vi "RAMP_init_ramp_scan.vi"(0 "queue CAMERA":refnum<queue>, 1 "queue piezo":refnum<queue>, 2 "queue DAQ":refnum<queue>, 3 "queue ASI stage":refnum<queue>, 4 "Laser lines array":dbl[][](array[numeric]), 5 "error in":errorcluster, 6 "Illumination source":bool, 7 "Brightfield intensity":dbl, 8 "Autofocus":bool, 9 "Movie path":path, 10 "Total range (nm)":u32=2000, 11 "z step (nm)":u32=50, 12 "Start acquisition":bool, 13 "Exp time (s)":sgl=0.05 format="%#_3g") -> (14 "Ramp":dbl[](array[numeric]), 16 "Total # z steps":i32, 17 "Ready":bool, 19 "error out":errorcluster)   [LabVIEW 2015]
uses:
  CONTROLS/Q_MCL_piezo_element.ctl
  CONTROLS/Q_camera_element.ctl
  CONTROLS/Q_ASI_stage_element.ctl
  CONTROLS/Q_DAQ_element.ctl
  GLOBAL/Global_DAQ.vi
  GLOBAL/Global_ASI_stage.vi
  GLOBAL/Global_MCL_piezo.vi
  GLOBAL/Global_CAMERA.vi
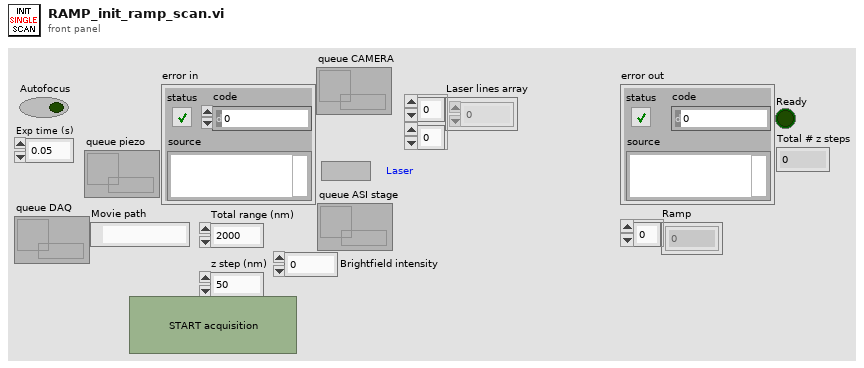
[diagram p1: front panel]
types:
  T1 = cluster{"Frames":i32, "Movie path":path, "Start acquisition":bool}
  T2 = typedef "Q_DAQ_element.ctl" = cluster{"variant":variant, "Instruction":enum16{"DAQ_idle", "DAQ_initialize", "DAQ_error", "DAQ_security_stop", "DAQ_start_QPD", "DAQ_change_QPD_display", "DAQ_read_display_QPD_signal", "DAQ_QPD_init_autofocus", "DAQ_read_display_send_QPD_signal", "DAQ_close_autofocus_calibration_ramp", "DAQ_close_autofocus", "DAQ_405", "DAQ_488", "DAQ_561", "DAQ_641", "DAQ_zero_all", "DAQ_init_single_scan", "DAQ_single_scan", "DAQ_two_way_valve", "DAQ_init_merFISH", "DAQ_scan_merFISH", "DAQ_photobleaching_merFISH", "DAQ_close_merFISH", "DAQ_stop"}}
  T3 = typedef "Q_camera_element.ctl" = cluster{"variant":variant, "Instruction":enum16{"CAMERA_idle", "CAMERA_initialize", "CAMERA_error", "CAMERA_security_stop", "CAMERA_not_acquiring", "CAMERA_acquiring", "CAMERA_start_acquiring", "CAMERA_stop_acquiring", "CAMERA_change_exposure", "CAMERA_define_ROI", "CAMERA_cooler", "CAMERA_acquire_movie", "CAMERA_init_scan", "CAMERA_check_new_scan_image", "CAMERA_close_scan", "CAMERA_init_merFISH", "CAMERA_start_acquiring_merFISH", "CAMERA_close_scan_merFISH", "CAMERA_close_merFISH", "CAMERA_init_TL", "CAMERA_start_acquiring_TL", "CAMERA_stop_acquiring_TL", "CAMERA_close_TL", "CAMERA_STOP"}}
  T4 = typedef "Q_MCL_piezo_element.ctl" = cluster{"variant":variant, "Instruction":enum16{"Piezo_idle", "Piezo_initialize", "Piezo_error", "Piezo_security_stop", "Piezo_read_z", "Piezo_move_z", "Piezo_keyboard_move", "Piezo_close_autofocus_calibration_ramp", "Piezo_change_init_state", "Piezo_init_autofocus", "Piezo_init_autofocus_merFISH_TL", "Piezo_autofocus", "Piezo_autofocus_merFISH_TL", "Piezo_stop_autofocus", "Piezo_stop_autofocus_merFISH_TL", "Piezo_autofocus_lost", "Piezo_resume_autofocus_merFISH_TL", "Piezo_check_z_position_merFISH_TL", "Piezo_init_ramp", "Piezo_move_z_ramp", "Piezo_close_ramp", "Piezo_close_merFISH", "Piezo_stop"}}
  T5 = cluster{"Illumination source":bool, "Laser lines array":dbl[][], "Exp time (s)":sgl}
  T6 = typedef "Q_ASI_stage_element.ctl" = cluster{"variant":variant, "Instruction":enum16{"ASI_idle", "ASI_initialize", "ASI_error", "ASI_security_stop", "ASI_read_XYZ", "ASI_up", "ASI_down", "ASI_left", "ASI_right", "ASI_save_XY", "ASI_move_to_XY", "ASI_brightfield", "ASI_init_scan", "ASI_init_merFISH", "ASI_move_to_XY_merFISH", "ASI_move_to_Z_merFISH", "ASI_init_autofocus_search_merFISH", "ASI_close_autofocus_search_merFISH", "ASI_adjust_piezo_autofocus_merFISH", "ASI_set_piezo_autofocus_to_reference_position_merFISH_TL", "ASI_close_merFISH", "ASI_stop"}}
  T7 = enum16{"DAQ_idle", "DAQ_initialize", "DAQ_error", "DAQ_security_stop", "DAQ_start_QPD", "DAQ_change_QPD_display", "DAQ_read_display_QPD_signal", "DAQ_QPD_init_autofocus", "DAQ_read_display_send_QPD_signal", "DAQ_close_autofocus_calibration_ramp", "DAQ_close_autofocus", "DAQ_405", "DAQ_488", "DAQ_561", "DAQ_641", "DAQ_zero_all", "DAQ_init_single_scan", "DAQ_single_scan", "DAQ_two_way_valve", "DAQ_init_merFISH", "DAQ_scan_merFISH", "DAQ_photobleaching_merFISH", "DAQ_close_merFISH", "DAQ_init_TL", "DAQ_synchro_TL", "DAQ_close_task_TL", "DAQ_close_TL", "DAQ_stop"}
  T8 = enum16{"DAQ_idle", "DAQ_initialize", "DAQ_error", "DAQ_security_stop", "DAQ_start_QPD", "DAQ_change_QPD_display", "DAQ_read_display_QPD_signal", "DAQ_QPD_init_autofocus", "DAQ_read_display_send_QPD_signal", "DAQ_close_autofocus_calibration_ramp", "DAQ_close_autofocus", "DAQ_405", "DAQ_488", "DAQ_561", "DAQ_641", "DAQ_zero_all", "DAQ_init_single_scan", "DAQ_single_scan", "DAQ_two_way_valve", "DAQ_init_merFISH", "DAQ_scan_merFISH", "DAQ_photobleaching_merFISH", "DAQ_close_merFISH", "DAQ_stop"}
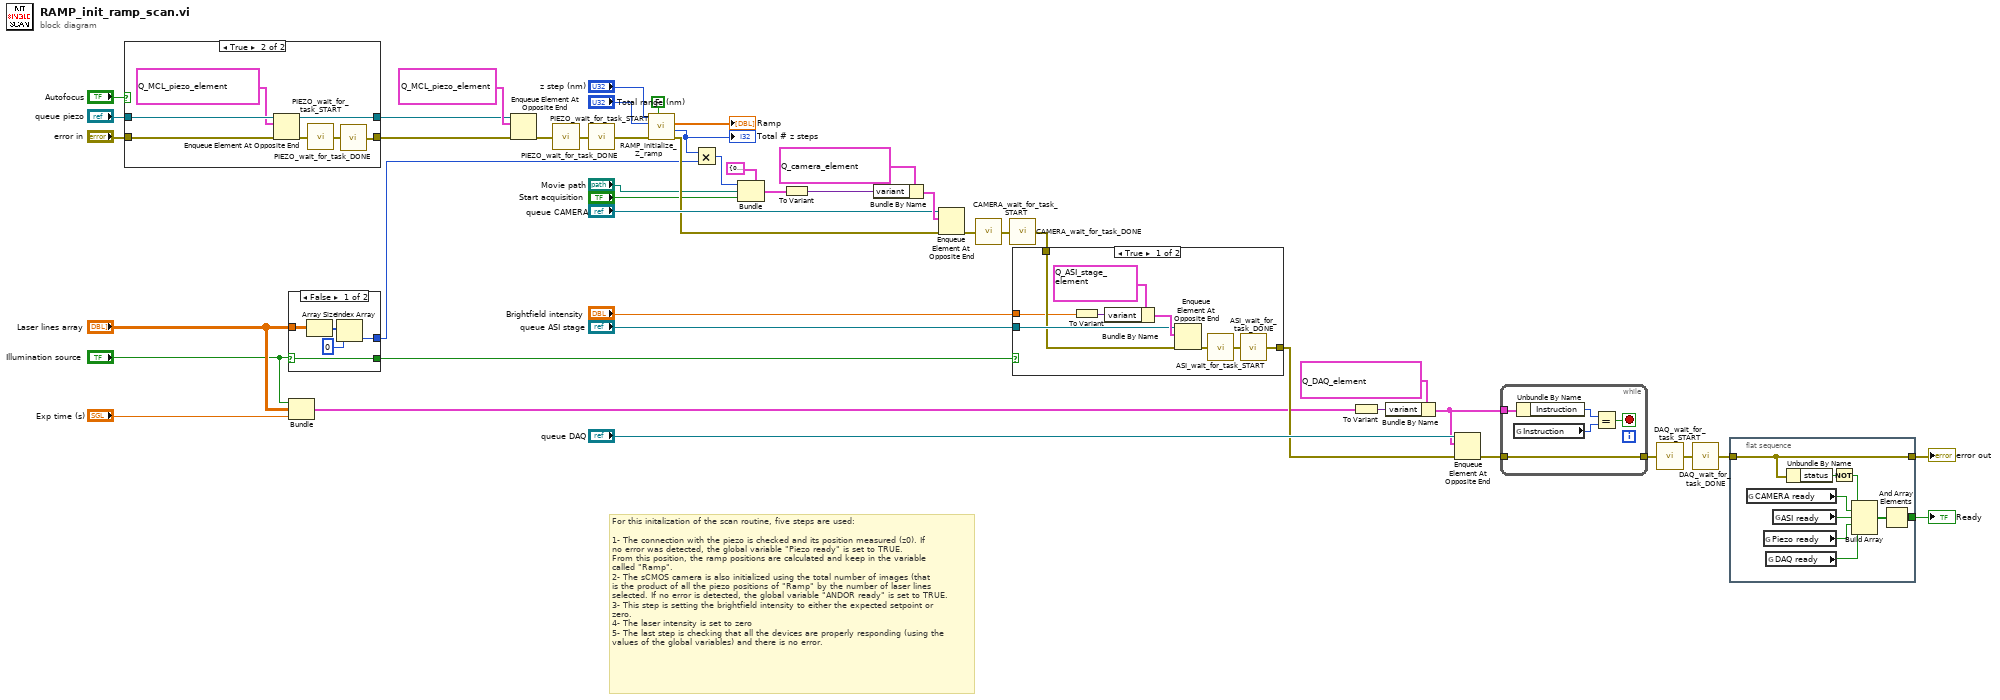
[diagram p0: block diagram]
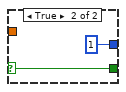
[diagram p2: hidden frame]
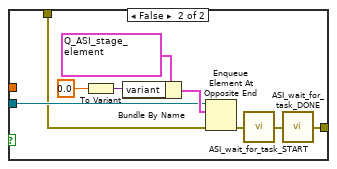
[diagram p4: hidden frame]
diagram:
  # "For this initalization of the scan routine, five steps are used:\n\n1- The connection with the piezo is checked and its position measured (z0). If\nno error was detected, the global variable \"Piezo ready\" is set to TRUE.\nFrom this position, the ramp positions are calculated and keep in the variable \ncalled \"Ramp\".\n2- The sCMOS camera is also initialized using the total number of images (that\nis the product of all the piezo positions of \"Ramp\" by the number of laser lines\nselected. If no error is detected, the global variable \"ANDOR ready\" is set to TRUE.\n3- This step is setting the brightfield intensity to either the expected setpoint or\nzero.\n4- The laser intensity is set to zero\n5- The last step is checking that all the devices are properly responding (using the\nvalues of the global variables) and there is no error."
  n1 = case shown="True" "Autofocus" {
    tunnel: "queue piezo" -> [w47 w55]
    tunnel: [w47 w54] -> w17
    tunnel: "error in" -> [w48 w52]
    tunnel: [w48 w49] -> w15
    frame False {
    }
    frame True {
      n2 = Enqueue Element At Opposite End(queue=w55, element=T4 {"variant"=variant, "Instruction"=enum."Piezo_stop_autofocus"}, error in (no error)=w52) -> (queue out=w54:refnum<queue>, error out=w51:errorcluster)  [unwired: 1 in, 1 out]
      n3 = call "PIEZO_wait_for_task_START.vi"("error in"=w51) -> ("error out"=w50:errorcluster)
      n4 = call "PIEZO_wait_for_task_DONE.vi"("error in"=w50) -> ("error out"=w49:errorcluster)
    }
  }
  n5 = case shown="False" "Illumination source" {
    selector: "Illumination source" -> [w56 w61]
    tunnel: "Laser lines array" -> [w60 _]
    tunnel: [w59 1] -> w10
    tunnel: [w56 w61] -> w11
    frame False {
      n6 = Array Size(array=w60) -> (size(s)=w58:i32[])
      n7 = Index Array(array=w58, index=0) -> (element=w59:i32)
    }
    frame True {
    }
  }
  n8 = Bundle("Illumination source"="Illumination source", "Laser lines array"="Laser lines array", "Exp time (s)"="Exp time (s)") -> (w5:T5)  [unwired: 1 in]
  n9 = Enqueue Element At Opposite End(queue=w17, element=T4 {"variant"=variant, "Instruction"=enum."Piezo_init_ramp"}, error in (no error)=w15) -> (error out=w46:errorcluster)  [unwired: 1 in, 2 out]
  n10 = call "PIEZO_wait_for_task_START.vi"("error in"=w46) -> ("error out"=w45:errorcluster)
  n11 = call "PIEZO_wait_for_task_DONE.vi"("error in"=w45) -> ("error out"=w43:errorcluster)
  n12 = call "RAMP_initialize_Z_ramp.vi"("Symmetric"=FALSE, "error in"=w43, "Total range (nm)"="Total range (nm)", "dZ (nm)"="z step (nm)") -> ("error out"=w37:errorcluster, "Total # steps"=w36:i32, "Ramp"=→"Ramp":dbl[])  [unwired: 1 in, 1 out]
  "Total # z steps" <- w36
  n13 = Multiply(x=w36, y=w10) -> (x*y=w14:i32)
  n14 = Bundle(cluster=T1 {"Frames"=0, "Movie path"=path "", "Start acquisition"=FALSE} ("output cluster"), "Frames"=w14, "Movie path"="Movie path", "Start acquisition"="Start acquisition") -> (w34:T1)
  n15 = To Variant(anything=w34) -> (Variant=w40:variant)
  n16 = Bundle By Name(cluster=T3 {"variant"=variant, "Instruction"=enum."CAMERA_init_scan"} ("Q_ANDOR_element"), "variant"=w40) -> (w39:T3)
  n17 = Enqueue Element At Opposite End(queue="queue CAMERA", element=w39, error in (no error)=w37) -> (error out=w33:errorcluster)  [unwired: 1 in, 2 out]
  n18 = call "CAMERA_wait_for_task_START.vi"("error in"=w33) -> ("error out"=w32:errorcluster)
  n19 = call "CAMERA_wait_for_task_DONE.vi"("error in"=w32) -> ("error out"=w31:errorcluster)
  n20 = case shown="True" w11 {
    tunnel: w31 -> [w67 w76]
    tunnel: "Brightfield intensity" -> [w63 _]
    tunnel: "queue ASI stage" -> [w68 w77]
    tunnel: [w64 w73] -> w24
    frame True {
      n21 = To Variant(anything=w63) -> (Variant=w70:variant)
      n22 = Bundle By Name(cluster=T6 {"variant"=variant, "Instruction"=enum."ASI_init_scan"} ("Q_ASI_stage"), "variant"=w70) -> (w69:T6)
      n23 = Enqueue Element At Opposite End(queue=w68, element=w69, error in (no error)=w67) -> (error out=w66:errorcluster)  [unwired: 1 in, 2 out]
      n24 = call "ASI_wait_for_task_START.vi"("error in"=w66) -> ("error out"=w65:errorcluster)
      n25 = call "ASI_wait_for_task_DONE.vi"("error in"=w65) -> ("error out"=w64:errorcluster)
    }
    frame False {
      n26 = To Variant(anything=0.0 ("Brightfield intensity")) -> (Variant=w79:variant)
      n27 = Bundle By Name(cluster=T6 {"variant"=variant, "Instruction"=enum."ASI_init_scan"} ("Q_ASI_stage"), "variant"=w79) -> (w78:T6)
      n28 = Enqueue Element At Opposite End(queue=w77, element=w78, error in (no error)=w76) -> (error out=w75:errorcluster)  [unwired: 1 in, 2 out]
      n29 = call "ASI_wait_for_task_START.vi"("error in"=w75) -> ("error out"=w74:errorcluster)
      n30 = call "ASI_wait_for_task_DONE.vi"("error in"=w74) -> ("error out"=w73:errorcluster)
    }
  }
  n31 = To Variant(anything=w5) -> (Variant=w8:variant)
  n32 = Bundle By Name(cluster=T2 {"variant"=variant, "Instruction"=enum."DAQ_init_single_scan"} ("Q_DAQ"), "variant"=w8) -> (w1:T2)
  n33 = Enqueue Element At Opposite End(queue="queue DAQ", element=w1, error in (no error)=w24) -> (error out=w3:errorcluster)  [unwired: 1 in, 2 out]
  n34 = while {
    tunnel: w3 -> [w82]
    tunnel: [w82] -> w2
    tunnel: w1 -> [w81]
    stop <- w84 stop-if-true
    n35 = global read "Global_DAQ.vi" "Instruction"() -> (w85:T7)
    n36 = Unbundle By Name(w81) -> ("Instruction"=w83:T8)
    n37 = Equal?(x=w83, y=w85) -> (x = y?=w84:bool)
  }
  n38 = call "DAQ_wait_for_task_START.vi"("error in"=w2) -> ("error out"=w23:errorcluster)
  n39 = call "DAQ_wait_for_task_DONE.vi"("error in"=w23) -> ("error out"=w22:errorcluster)
  n40 = flat-sequence {
    tunnel: [w94] -> w20
    tunnel: w22 -> [w87]
    tunnel: [w87] -> w21
    frame #0 {
      n41 = global read "Global_CAMERA.vi" "CAMERA ready"() -> (w91:bool)
      n42 = global read "Global_MCL_piezo.vi" "Piezo ready"() -> (w92:bool)
      n43 = global read "Global_DAQ.vi" "DAQ ready"() -> (w86:bool)
      n44 = global read "Global_ASI_stage.vi" "ASI ready"() -> (w93:bool)
      n45 = Unbundle By Name(w87) -> ("status"=w89:bool)
      n46 = Not(x=w89) -> (.not. x?=w88:bool)
      n47 = Build Array(w88, w91, w93, w92, w86) -> (w90:bool[])
      n48 = And Array Elements(Boolean array=w90) -> (logical AND=w94:bool)
    }
  }
  "error out" <- w21
  "Ready" <- w20
